vi "Close.vi"(8 "error in (no error)":errorcluster, 11 "VISA resource name":refnum<visa-resource-name>) -> (0 "error out":errorcluster)   [LabVIEW 2017, in "Digikrom DK24x.lvlib"]
doc: "Closes all handles associated with the instrument."
uses:
  Digikrom DK24x.lvlib
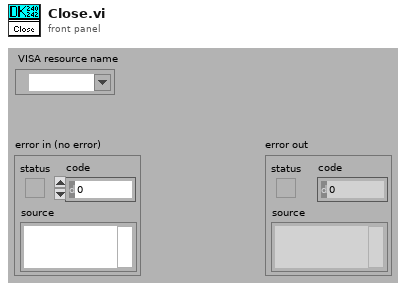
[diagram p1: front panel]
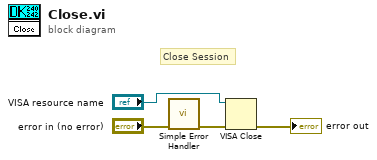
[diagram p0: block diagram]
diagram:
  # "Close Session"
  n1 = call <vilib>:"Simple Error Handler.vi"("error in (no error)"="error in (no error)") -> ("error out"=w2:errorcluster)  [unwired: 1 in, 7 out]
  n2 = VISA Close(VISA resource name="VISA resource name", error in (no error)=w2) -> (error out=→"error out":errorcluster)
